vi "compliancevi3subvi.vi"(0 "compliance (A)":dbl=0.0001 format="%^.2e", 4 "start":dbl, 5 "compliance (V)":dbl=0.0001 format="%^.2e", 6 "total points":u16, 7 "step":dbl, 8 "Mode":u16(ring)=4 items=["V", "I", "VPulse", "IPulse", "Common"], 9 "Value1":dbl) -> (1 "total points 2":u16, 2 "compliance":dbl, 3 "constant":dbl)   [LabVIEW 2012]
uses:
  Instance           1 26Saved   compliancevi3subvi .vi
  Instance           2 26Saved   compliancevi3subvi .vi
  Instance           3 26Saved   compliancevi3subvi .vi
  Instance           4 26Saved   compliancevi3subvi .vi
  Instance           5 26Saved   compliancevi3subvi .vi
  Instance           6 26Saved   compliancevi3subvi .vi
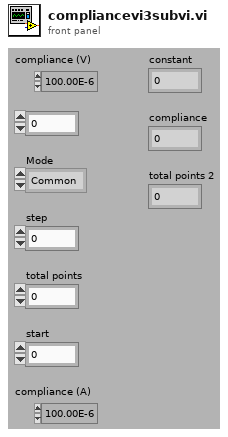
[diagram p1: front panel]
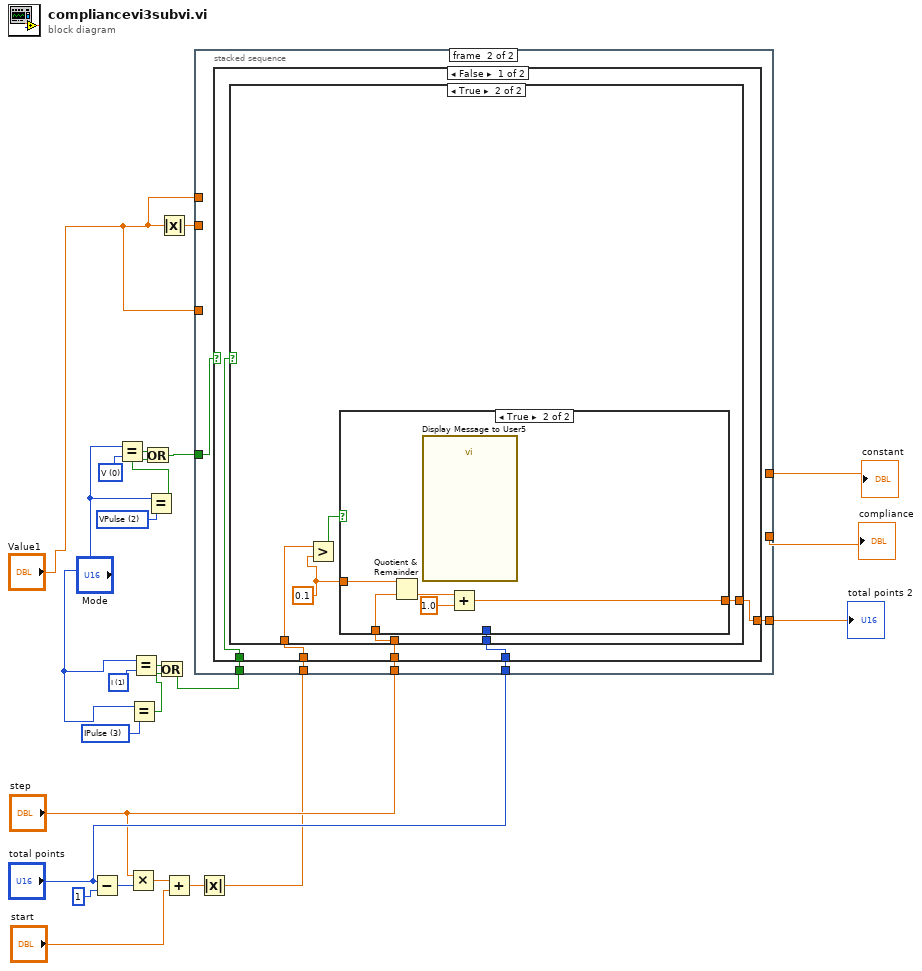
[diagram p0: block diagram]
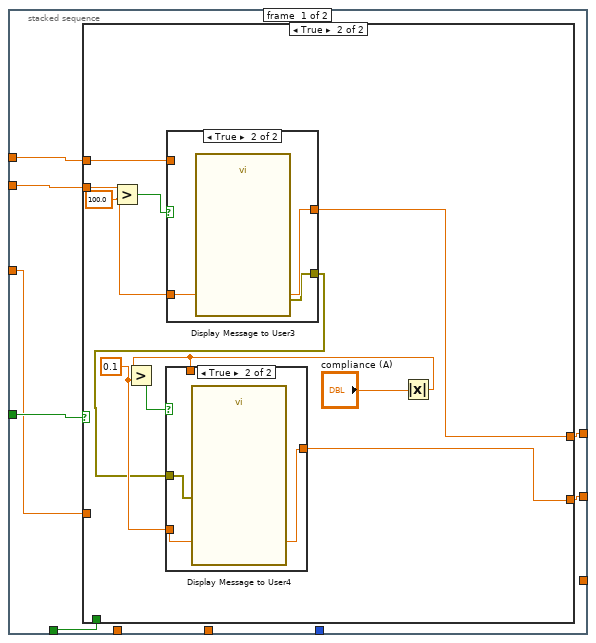
[diagram p2: hidden frame]
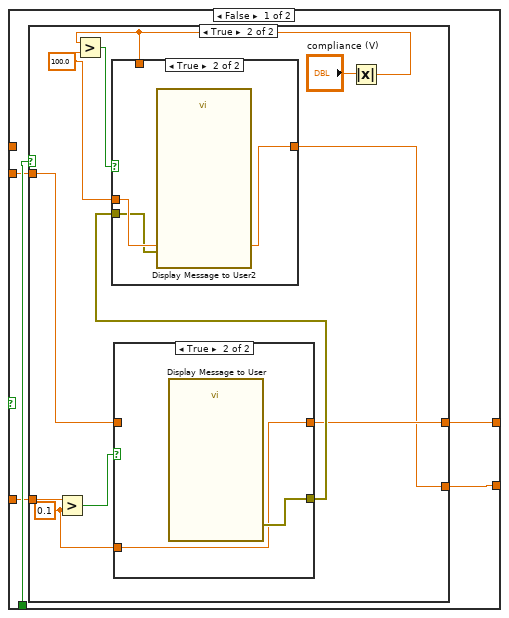
[diagram p3: hidden frame]
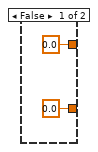
[diagram p4: hidden frame]
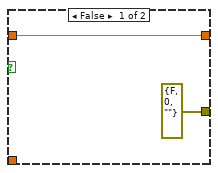
[diagram p5: hidden frame]
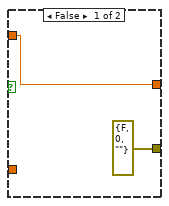
[diagram p7: hidden frame]
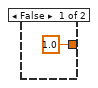
[diagram p9: hidden frame]
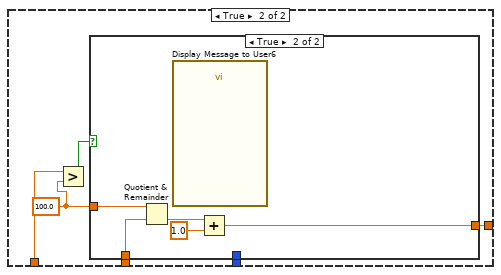
[diagram p11: hidden frame]
diagram:
  w3 = u16 3 items=["V", "I", "VPulse", "IPulse", "Common"] ("Mode")
  w4 = u16 1 items=["V", "I", "VPulse", "IPulse", "Common"] ("Mode")
  w9 = u16 2 items=["V", "I", "VPulse", "IPulse", "Common"] ("Mode")
  w11 = u16 0 items=["V", "I", "VPulse", "IPulse", "Common"] ("Mode")
  n1 = Subtract(x="total points", y=u16 1) -> (x-y=w16:u16)
  n2 = Equal?(x="Mode", y=w11) -> (x = y?=w10:bool)
  n3 = Multiply(x="step", y=w16) -> (x*y=w17:dbl)
  n4 = Equal?(x="Mode", y=w3) -> (x = y?=w5:bool)
  n5 = Equal?(x="Mode", y=w4) -> (x = y?=w6:bool)
  n6 = Equal?(x="Mode", y=w9) -> (x = y?=w8:bool)
  n7 = Or(x=w10, y=w8) -> (x .or. y?=w7:bool)
  n8 = Or(x=w6, y=w5) -> (x .or. y?=w12:bool)
  n9 = Absolute Value(x="Value1") -> (abs(x)=w1:dbl)
  n10 = Add(x=w17, y="start") -> (x+y=w19:dbl)
  n11 = Absolute Value(x=w19) -> (abs(x)=w21:dbl)
  n12 = stacked-sequence {
    tunnel: w1 -> [w31 _]
    tunnel: w7 -> [w30 w80]
    tunnel: w12 -> [w29 w75]
    tunnel: "Value1" -> [w28 _]
    tunnel: [w27 _] -> w13
    tunnel: [w26 _] -> w14
    tunnel: "Value1" -> [w25 _]
    tunnel: w21 -> [_ w79]
    tunnel: "step" -> [_ w78]
    tunnel: [_ w77] -> w23
    tunnel: "total points" -> [_ w76]
    frame #0 {
      n13 = case shown="True" w30 {
        tunnel: w31 -> [w35 w63]
        tunnel: w28 -> [_ w60]
        tunnel: w29 -> [w36 _]
        tunnel: w25 -> [w34 _]
        tunnel: [w33 w58] -> w27
        tunnel: [w32 w57] -> w26
        frame False {
          n14 = case shown="True" w36 {
            tunnel: w34 -> [_ w45]
            tunnel: w35 -> [_ w41]
            tunnel: [0.0 ("y") w40] -> w33
            tunnel: [0.0 ("y") w39] -> w32
            frame False {
            }
            frame True {
              w42 = 0.1 ("y")
              w48 = 100.0 ("y")
              n15 = Greater?(x=w45, y=w42) -> (0:w44:bool)
              n16 = case shown="True" w44 {
                tunnel: [errorcluster {"status"=FALSE, "code"=0, "source"=""} ("error out") w53] -> w43
                tunnel: [w50 w52] -> w40
                tunnel: w41 -> [w50 _]
                tunnel: w42 -> [_ w52]
                frame False {
                }
                frame True {
                  n17 = call "Display Message to User"() -> ("error out"=w53:errorcluster)  [unwired: 10 in, 1 out]
                }
              }
              n18 = Absolute Value(x="compliance (V)") -> (abs(x)=w46:dbl)
              n19 = Greater?(x=w46, y=w48) -> (0:w49:bool)
              n20 = case shown="True" w49 {
                tunnel: w46 -> [w54 _]
                tunnel: w48 -> [_ w56]
                tunnel: [w54 w56] -> w39
                tunnel: w43 -> [_ w55]
                frame False {
                }
                frame True {
                  n21 = call "Display Message to User2"("error in (no error)"=w55) -> ()  [unwired: 9 in, 2 out]
                }
              }
            }
          }
        }
        frame True {
          w61 = 100.0 ("y")
          w66 = 0.1 ("y")
          n22 = Greater?(x=w63, y=w61) -> (0:w62:bool)
          n23 = case shown="True" w62 {
            tunnel: w61 -> [_ w71]
            tunnel: [w69 w71] -> w58
            tunnel: w60 -> [w69 _]
            tunnel: [errorcluster {"status"=FALSE, "code"=0, "source"=""} ("error out") w70] -> w59
            frame False {
            }
            frame True {
              n24 = call "Display Message to User3"() -> ("error out"=w70:errorcluster)  [unwired: 10 in, 1 out]
            }
          }
          n25 = Absolute Value(x="compliance (A)") -> (abs(x)=w64:dbl)
          n26 = Greater?(x=w64, y=w66) -> (0:w67:bool)
          n27 = case shown="True" w67 {
            tunnel: w66 -> [_ w74]
            tunnel: [w72 w74] -> w57
            tunnel: w64 -> [w72 _]
            tunnel: w59 -> [_ w73]
            frame False {
            }
            frame True {
              n28 = call "Display Message to User4"("error in (no error)"=w73) -> ()  [unwired: 9 in, 2 out]
            }
          }
        }
      }
    }
    frame #1 {
      n29 = case shown="False" w80 {
        tunnel: w79 -> [w84 w104]
        tunnel: w78 -> [w83 w101]
        tunnel: [w81 w100] -> w77
        tunnel: w76 -> [w82 w99]
        tunnel: w75 -> [w85 _]
        frame False {
          n30 = case shown="True" w85 {
            tunnel: w84 -> [_ w90]
            tunnel: w83 -> [_ w89]
            tunnel: w82 -> [_ w88]
            tunnel: [1.0 ("total points") w87] -> w81
            frame False {
            }
            frame True {
              w91 = 0.1 ("y")
              n31 = Greater?(x=w90, y=w91) -> (0:w92:bool)
              n32 = case shown="True" w92 {
                tunnel: w91 -> [_ w98]
                tunnel: w89 -> [_ w97]
                tunnel: [w93 w94] -> w87
                tunnel: w88 -> [w93 _]
                frame False {
                }
                frame True {
                  n33 = Quotient & Remainder(x=w98, y=w97) -> (floor(x/y)=w96:dbl)  [unwired: 1 out]
                  n34 = call "Display Message to User5"() -> ()  [unwired: 10 in, 2 out]
                  n35 = Add(x=w96, y=1.0) -> (x+y=w94:dbl)
                }
              }
            }
          }
        }
        frame True {
          w102 = 100.0 ("y")
          n36 = Greater?(x=w104, y=w102) -> (0:w103:bool)
          n37 = case shown="True" w103 {
            tunnel: w102 -> [_ w110]
            tunnel: w101 -> [_ w109]
            tunnel: [w105 w106] -> w100
            tunnel: w99 -> [w105 _]
            frame False {
            }
            frame True {
              n38 = Quotient & Remainder(x=w110, y=w109) -> (floor(x/y)=w108:dbl)  [unwired: 1 out]
              n39 = call "Display Message to User6"() -> ()  [unwired: 10 in, 2 out]
              n40 = Add(x=w108, y=1.0) -> (x+y=w106:dbl)
            }
          }
        }
      }
    }
  }
  "compliance" <- w14
  "constant" <- w13
  "total points 2" <- w23
